vi "Test Case.Serialize - Invalid character in Type - XML does not contain invalid character.vi"() -> ()   [LabVIEW 2013, in "JUnit XML Tests.lvlib"]
uses:
  JUnit XML Tests.lvlib
  <vilib>/xml/Close Reference(Node).vi
  <vilib>/addons/_JKI Toolkits/Caraya/classes/Assert/Assert Equal Value_Variant.vi
  JUnit XML/JUnit XML.lvlib
  <vilib>/addons/_JKI Toolkits/Caraya/classes/Test/Test.lvclass
  <vilib>/addons/_JKI Toolkits/Caraya/classes/Assert/Assert.lvclass
  <resource>/objmgr/DOMUserDefRef.rc
  <vilib>/xml/NI_XML.lvlib
  JUnit XML/Test Case/Test Case.lvclass
panel:
  out "error out":errorcluster
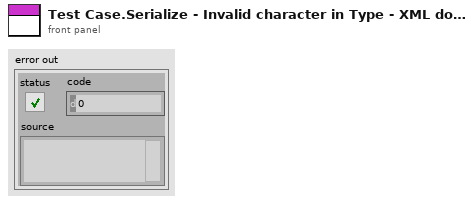
[diagram p1: front panel]
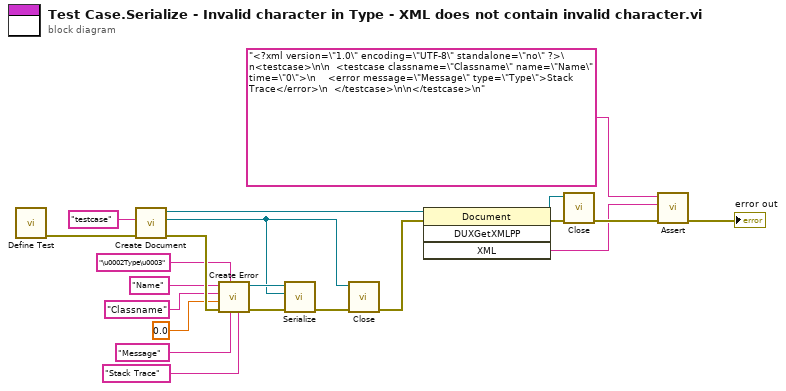
[diagram p0: block diagram]
diagram:
  n1 = call <vilib>:"Define Test.vi"() -> ("error out"=w21:errorcluster)  [unwired: 10 in, 1 out]
  n2 = call "Create Document.vi"("error in (no error)"=w21, "Root Element Name"="testcase") -> ("error out"=w17:errorcluster, "Root Element"=w13:refnum<k20>, "Document"=w16:refnum<k20>)  [unwired: 7 in]
  n3 = call "Create Error.vi"("Stack Trace"="Stack Trace", "Message"="Message", "Type"="\u0002Type\u0003", "error in (no error)"=w17, "Time"=0.0, "Classname"="Classname", "Name"="Name") -> ("error out"=w19:errorcluster, "Test Case"=w20:refnum<class "Test Case.lvclass">)  [unwired: 3 in]
  n4 = call "Serialize.vi"("error in (no error)"=w19, "Element in"=w13, "Test Case in"=w20) -> ("error out"=w15:errorcluster)  [unwired: 7 in, 1 out]
  n5 = call-poly <vilib>:"Close.vi"("error in (no error)"=w15, "node"=w13) -> ("error out"=w14:errorcluster)  [unwired: 7 in]
  n6 = invoke class="Document" method="DUXGetXMLPP"(reference=w16, error in=w14) -> (reference out=w11:refnum<k20>, error out=w12:errorcluster, "XML"=w9:string)  [unwired: 2 in, 1 out]
  n7 = call-poly <vilib>:"Close.vi"("error in (no error)"=w12, "node"=w11) -> ("error out"=w10:errorcluster)  [unwired: 7 in]
  n8 = call-poly <vilib>:"Assert.vi"("error in (no error)"=w10, "Actual"=w9, "Expected"="<?xml version=\"1.0\" encoding=\"UTF-8\" standalone=\"no\" ?>\n<testcase>\n\n  <testcase classname=\"Classname\" name=\"Name\" time=\"0\">\n    <error message=\"Message\" type=\"Type\">Stack Trace</error>\n  </testcase>\n\n</testcase>\n") -> ("error out"=→"error out":errorcluster)  [unwired: 7 in, 1 out]
